vi "Close Device Core.vi"(8 "error in (no error)":errorcluster, 11 "KIT-QVA in":refnum<class "KIT-QVA.lvclass">) -> (0 "error out":errorcluster, 3 "KIT-QVA out":refnum<class "KIT-QVA.lvclass">)   [LabVIEW 2014, in "KIT-QVA.lvlib" / "KIT-QVA.lvclass"]
doc: "Close device driver connection."
uses:
  KIT-QVA.lvclass
  KIT-QVA.lvclass/KIT-QVA.ctl
  CSPP_Core/Actors/CS++DeviceActor/CS++DeviceActor.lvclass
  instr.lib/KIT-QV/KIT QV.lvlib
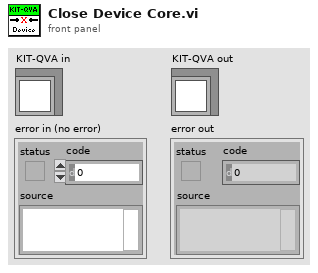
[diagram p1: front panel]
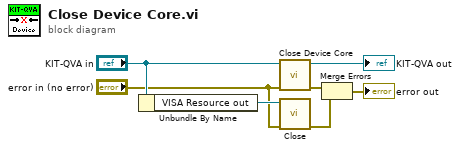
[diagram p0: block diagram]
diagram:
  n1 = Unbundle By Name("KIT-QVA in") -> ("VISA Resource out"=w4:refnum<visa-resource-name>)
  n2 = call-parent "Close Device Core.vi"("error in (no error)"="error in (no error)", "CS++DeviceActor in"="KIT-QVA in") -> ("error out"=w7:errorcluster, "CS++DeviceActor out"=→"KIT-QVA out":refnum<class "KIT-QVA.lvclass">)  [unwired: 8 in]
  n3 = call "Close.vi"("Error In"="error in (no error)", "VISA Resource in"=w4) -> ("Error Out"=w1:errorcluster)  [unwired: 9 in]
  n4 = Merge Errors(w7, w1) -> (→"error out":errorcluster)
